vi "Collate_Data.vi"(1 "Value in":dbl) -> (0 "Flow Out":dbl[](array[numeric]))   [LabVIEW 2014]
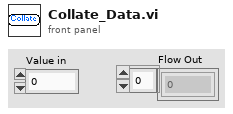
[diagram p1: front panel]
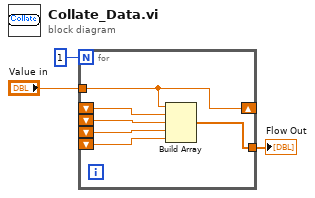
[diagram p0: block diagram]
diagram:
  n1 = for {
    N: 1 -> [_]
    tunnel: "Value in" -> [w5]
    shift-right: [w5] -> _
    shift-left: _ -> [w9]
    shift-left: _ -> [w8]
    tunnel: [w4] -> w1
    shift-left: _ -> [w7]
    shift-left: _ -> [w6]
    n2 = Build Array(w5, w9, w8, w7, w6) -> (w4:dbl[])
  }
  "Flow Out" <- w1
